vi "CRYUnflatten Custom.vi"(11 "Unflatten Custom":string) -> (0 "Error?":bool, 2 "Custom":T2, 3 "Header info":T1={"Data type"="Data            ", "Version"=1, "Dimensions"=0})   [LabVIEW 2013]
uses:
  Typedef Control/CRYCustom Cluster.ctl
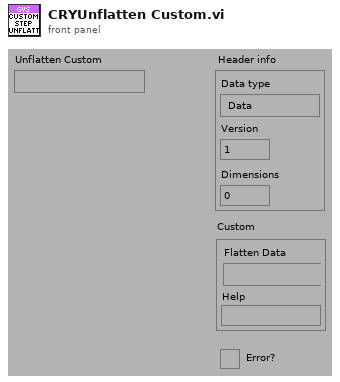
[diagram p1: front panel]
types:
  T1 = cluster{"Data type":string, "Version":u16, "Dimensions":u8}
  T2 = typedef "CRYCustom Cluster.ctl" = cluster{"Help":string, "Flatten Data":string}
  T3 = cluster{"unsigned byte array[0]":u8, "unsigned byte array[1]":u8, "unsigned byte array[2]":u8}
  T4 = cluster{"substring":string, u16, "unsigned byte array[2]":u8}
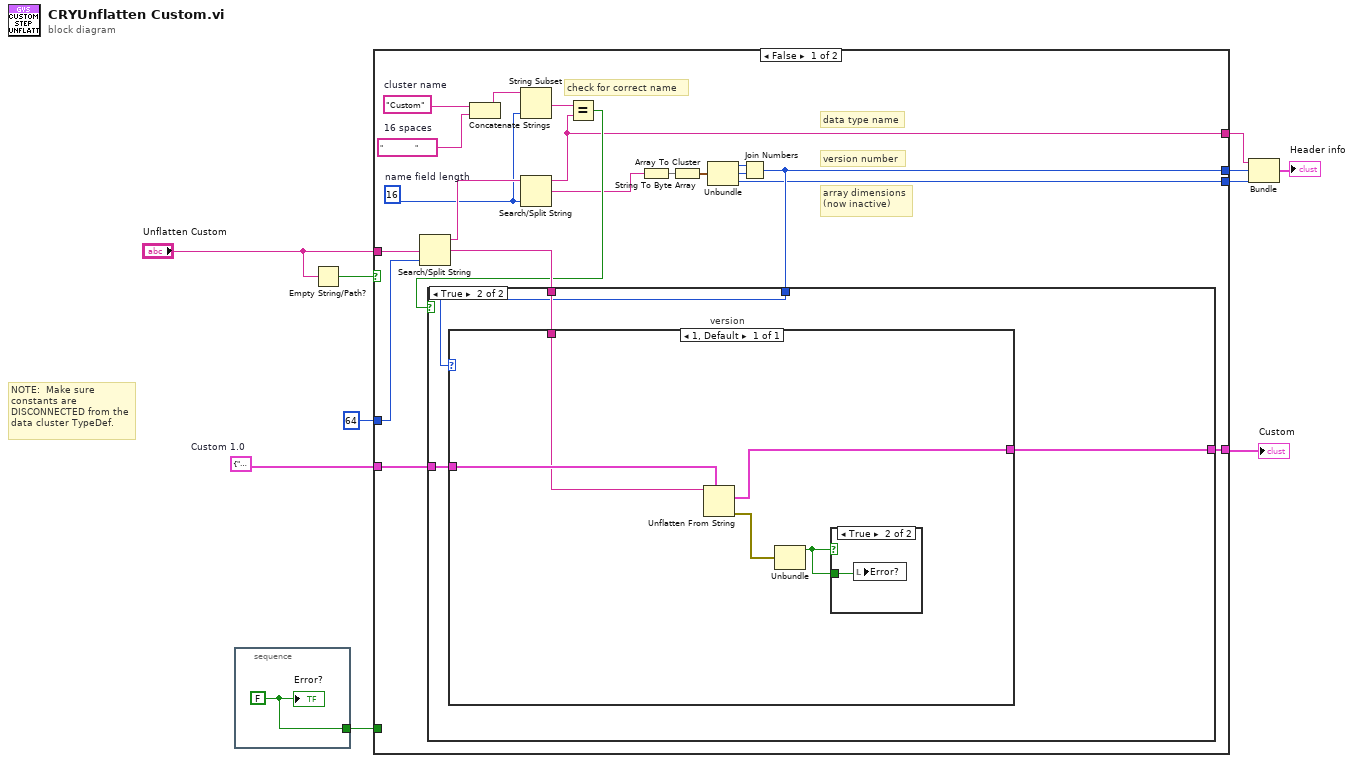
[diagram p0: block diagram]
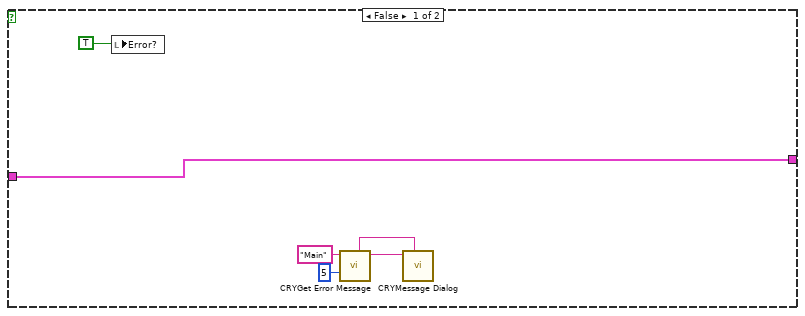
[diagram p2: hidden frame]
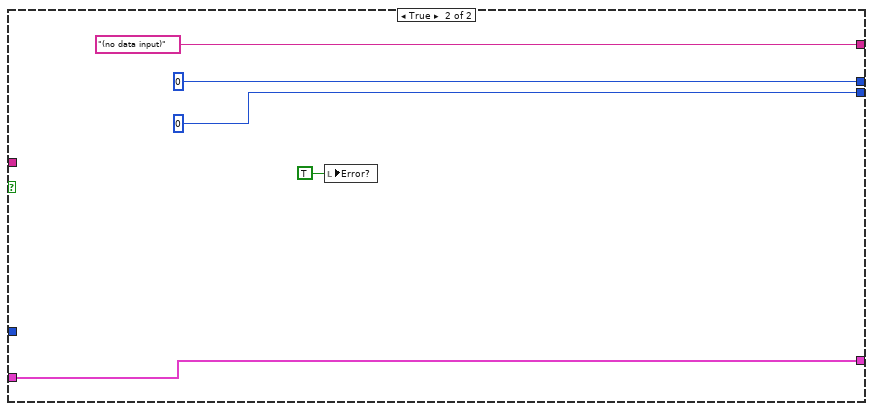
[diagram p4: hidden frame]
diagram:
  w1 = cluster{"Help":string, "Flatten Data":string} {"Help"="", "Flatten Data"=""}  # Custom 1.0
  # "NOTE:  Make sure constants are DISCONNECTED from the data cluster TypeDef."
  n1 = stacked-sequence {
    tunnel: [w11] -> w3
    frame #0 {
      w11 = FALSE
      "Error?" <- w11
    }
  }
  n2 = Empty String/Path?(string/path="Unflatten Custom") -> (empty?=w9:bool)
  n3 = case shown="False" w9 {
    tunnel: "Unflatten Custom" -> [w31 _]
    tunnel: 64 ("header length") -> [w25 _]
    tunnel: [w22 u16 0] -> w6
    tunnel: [w14 u8 0] -> w7
    tunnel: [w15 "(no data input)" ("substring")] -> w5
    tunnel: w3 -> [_ _]
    tunnel: [w13 w48] -> w2
    tunnel: w1 -> [w12 w48]
    frame False {
      w19 = "                "  # 16 spaces
      w20 = "Custom"  # cluster name
      w17 = 16  # name field length
      # "check for correct name"
      # "array dimensions\n(now inactive)"
      # "version number"
      # "data type name"
      n4 = Search/Split String(string=w31, offset (0)=w25) -> (substring before match=w24:string, match + rest of string=w26:string)  [unwired: 2 out]
      n5 = Concatenate Strings(w20, w19) -> (w18:string)
      n6 = String Subset(string=w18, length (rest)=w17) -> (substring=w16:string)  [unwired: 1 out]
      n7 = Search/Split String(string=w24, offset (0)=w17) -> (substring before match=w15:string, match + rest of string=w21:string)  [unwired: 2 out]
      n8 = Equal?(x=w16, y=w15) -> (x = y?=w23:bool)
      n9 = String To Byte Array(string=w21) -> (unsigned byte array=w30:u8[])
      n10 = Array To Cluster(array=w30) -> (cluster=w29:T3)
      n11 = Unbundle(w29) -> ("unsigned byte array[0]"=w28:u8, "unsigned byte array[1]"=w27:u8, "unsigned byte array[2]"=w14:u8)
      n12 = Join Numbers(hi=w28, lo=w27) -> ((hi.lo)=w22:u16)
      n13 = case shown="True" w23 {
        tunnel: w26 -> [_ w41]
        tunnel: w22 -> [_ w40]
        tunnel: [w36 w39] -> w13
        tunnel: w12 -> [w36 w38]
        frame False {
          n14 = local write "Error?"(TRUE) -> ()
          n15 = call "CRYGet Error Message.vi"("Error No"=5, "Kind"="Main") -> ("Message"=w33:string, "Window Title"=w32:string)  [unwired: 4 in, 4 out]
          n16 = call "CRYMessage Dialog.vi"("Window Title"=w32, "Message Content"=w33) -> ()  [unwired: 8 in, 2 out]
        }
        frame True {
          n17 = case "version" shown="1, Default" w40 {
            tunnel: w41 -> [w45]
            tunnel: [w44] -> w39
            tunnel: w38 -> [w46]
            frame 1, Default {
              n18 = Unflatten From String(type=w46, binary string=w45) -> (value=w44:cluster{"Help":string, "Flatten Data":string}, error out=w43:errorcluster)  [unwired: 1 in, 3 out]
              n19 = Unbundle(w43) -> ("status"=w42:bool)  [unwired: 2 out]
              n20 = case shown="True" w42 {
                tunnel: w42 -> [_ w47]
                frame False {
                }
                frame True {
                  n21 = local write "Error?"(w47) -> ()
                }
              }
            }
          }
        }
      }
    }
    frame True {
      n22 = local write "Error?"(TRUE ("Error?")) -> ()
    }
  }
  "Custom" <- w2
  n23 = Bundle("substring"=w5, w6, "unsigned byte array[2]"=w7) -> (→"Header info":T4)  [unwired: 1 out]
